vi "Receive and Display using Event Log.vi"() -> ()   [LabVIEW 2023]
uses:
  <instrlib>/BTICardLib/Public/Controls/Event Log Type.ctl
  <instrlib>/BTICardLib/Private/Initialize By Card Number and Core Number.vi
  <instrlib>/BTICardLib/Private/Configure Core From XML.vi
  <instrlib>/BTI429Lib/Private/Rx/Configure/Configure Rx Channel From XML.vi
  <instrlib>/BTI429Lib/Private/Rx/Configure/Get Rx Label Handle Name.vi
  <instrlib>/BTI429Lib/Private/Core/Action-Status/Start Channel.vi
  <instrlib>/BTI429Lib/Private/Core/Action-Status/Stop Channel.vi
  <instrlib>/BTICardLib/BTICardLV.lvlib
  <instrlib>/BTI429Lib/BTI429LV.lvlib
panel:
  out "CoreXml Path":path
  out "Channel Xml Path":path
  in  "Channel number":i32
  in  "core number":i32
  in  "Channel Configuration XML file name":string="Channel Config.xml"
  in  "Core Configuration XML file name":string="Core Config.xml"
  out "error out":errorcluster
  in  "Card Number":i32
  out "Data 2":u32 format="%x"
  out "Data 1":u32 format="%x"
  out "Default":u32 format="%x"
  in  "stop":bool
  # "ARINC 429: Receive Labels"
  # "©2016 Astronics Ballard Technology"
  # "The  message labels are read from the Channel Configuration XML file.\n\nThe label definitions enable Event Log Recording of Message actitivty. The \nEvent Log is polled for 429 Messages and when a specific label has been \nreceived, its data is updated on the front panel."
  # "Always Stop the card\nand Close the card when\ndone. Otherwise, the hardware\ncontinues to operate."
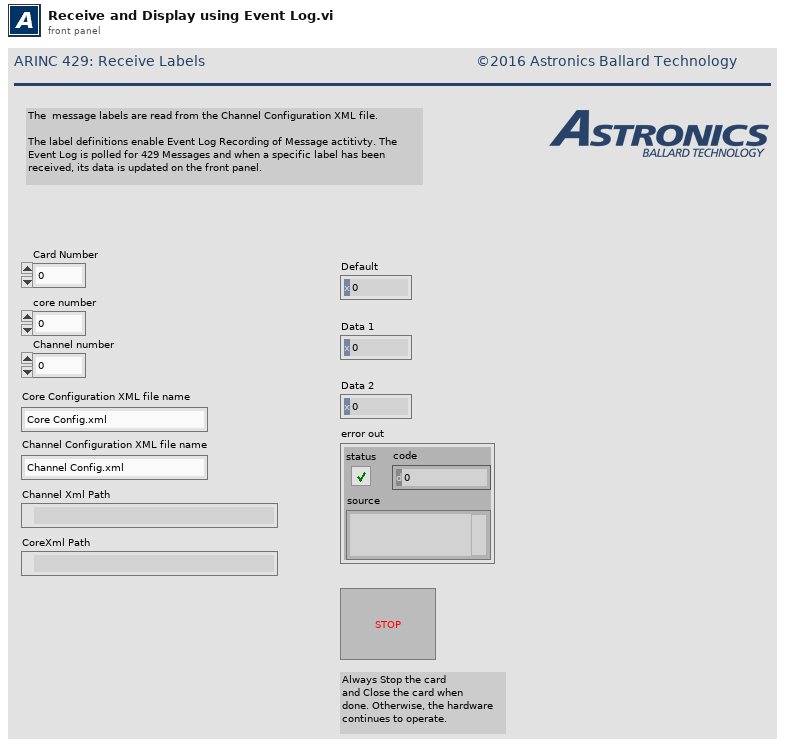
[diagram p1: front panel]
types:
  T1 = typedef "BTICardLV.lvlib/Event Log Type.ctl" = u32
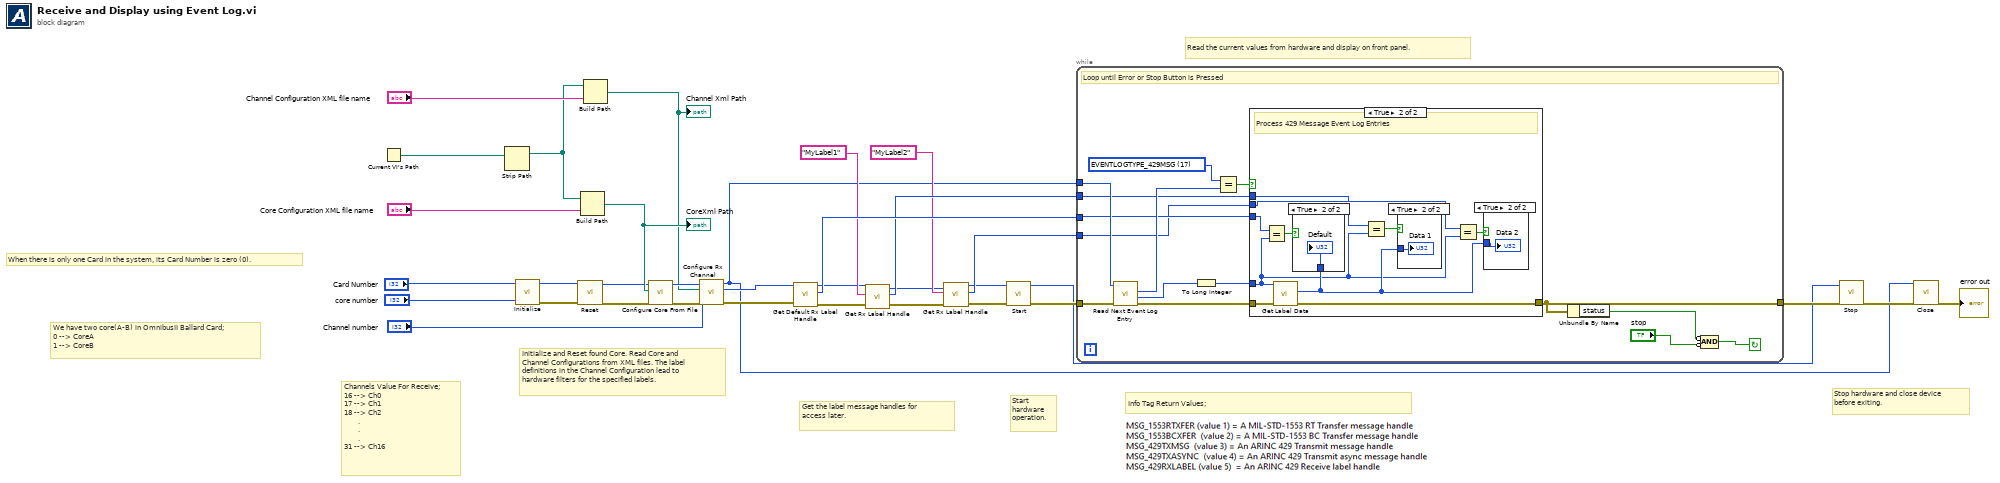
[diagram p0: block diagram]
diagram:
  # "We have two core(A-B) in OmnibusII Ballard Card;\n0 --> CoreA\n1 --> CoreB"
  # "When there is only one Card in the system, its Card Number is zero (0)."
  # "Channels Value For Receive;\n16 --> Ch0\n17 --> Ch1\n18 --> Ch2\n       .\n       .\n       .\n31 --> Ch16"
  # "Info Tag Return Values;"
  # "Stop hardware and close device\nbefore exiting."
  # "Read the current values from hardware and display on front panel."
  # "Start\nhardware\noperation."
  # "Get the label message handles for\naccess later."
  # "Initialize and Reset found Core. Read Core and\nChannel Configurations from XML files. The label\ndefinitions in the Channel Configuration lead to\nhardware filters for the specified labels."
  n1 = Current VI's Path() -> (path=w13:path)
  n2 = Strip Path(path=w13) -> (stripped path=w11:path)  [unwired: 1 out]
  n3 = call-poly <instrlib>:"Initialize.vi"("core number"="core number", "card number"="Card Number") -> ("error out"=w6:errorcluster, "core handle out"=w4:u64)  [unwired: 8 in]
  n4 = call <instrlib>:"Reset.vi"("error in (no error)"=w6, "core handle in"=w4) -> ("error out"=w5:errorcluster, "core handle out"=w3:u64)  [unwired: 8 in]
  n5 = Build Path(base path=w11, name or relative path="Core Configuration XML file name") -> (appended path=w9:path)
  "CoreXml Path" <- w9
  n6 = Build Path(base path=w11, name or relative path="Channel Configuration XML file name") -> (appended path=w8:path)
  "Channel Xml Path" <- w8
  n7 = call-poly <instrlib>:"Configure Core From File.vi"("error in (no error)"=w5, "configuration file path"=w9, "core handle in"=w3) -> ("error out"=w25:errorcluster, "core handle out"=w20:u64)  [unwired: 7 in]
  n8 = call-poly <instrlib>:"Configure Rx Channel.vi"("error in (no error)"=w25, "channel number in"="Channel number", "configuration file path"=w8, "core handle in"=w20) -> ("error out"=w34:errorcluster, "channel handle out"=w19:u64, "core handle out"=w18:u64)  [unwired: 5 in]
  n9 = call <instrlib>:"Get Default Rx Label Handle.vi"("error in (no error)"=w34, "channel handle in"=w19) -> ("error out"=w33:errorcluster, "default label handle out"=w29:u64, "channel handle out"=w17:u64)  [unwired: 7 in]
  n10 = call-poly <instrlib>:"Get Rx Label Handle.vi"("error in (no error)"=w33, "label name"="MyLabel1", "channel handle in"=w17) -> ("error out"=w32:errorcluster, "label handle out"=w28:u64, "channel handle out"=w16:u64)  [unwired: 6 in]
  n11 = call-poly <instrlib>:"Get Rx Label Handle.vi"("error in (no error)"=w32, "label name"="MyLabel2", "channel handle in"=w16) -> ("error out"=w31:errorcluster, "label handle out"=w27:u64, "channel handle out"=w15:u64)  [unwired: 6 in]
  n12 = call-poly <instrlib>:"Start.vi"("error in (no error)"=w31, "channel handle in"=w15) -> ("error out"=w30:errorcluster, "channel handle out"=w14:u64)  [unwired: 8 in]
  n13 = while {
    tunnel: w30 -> [w46]
    tunnel: w29 -> [w40]
    tunnel: w28 -> [w37]
    tunnel: w27 -> [w38]
    tunnel: [w39] -> w21
    tunnel: w18 -> [w44]
    stop <- w49 continue-if-true
    w42 = T1 17 items=["EVENTLOGTYPE_NONE"=0, "EVENTLOGTYPE_1553MSG"=1, "EVENTLOGTYPE_1553OPCODE"=2, "EVENTLOGTYPE_1553HALT"=3, "EVENTLOGTYPE_1553PAUSE"=4, "EVENTLOGTYPE_1553LIST"=5, "EVENTLOGTYPE_1553SERIAL"=6, "EVENTLOGTYPE_429MSG"=17, "EVENTLOGTYPE_429OPCODE"=18, "EVENTLOGTYPE_429HALT"=19, "EVENTLOGTYPE_429PAUSE"=20, "EVENTLOGTYPE_429LIST"=21, "EVENTLOGTYPE_429ERR"=22, "EVENTLOGTYPE_DIOEDGE"=96, "EVENTLOGTYPE_DIOFAULT"=97, "EVENTLOGTYPE_BITERROR"=113] ("x")
    # "Loop until Error or Stop Button is Pressed"
    n14 = call <instrlib>:"Read Next Event Log Entry.vi"("error in (no error)"=w46, "core handle in"=w44) -> ("error out"=w45:errorcluster, "info tag"=w35:u64, "event log entry type"=w43:T1)  [unwired: 4 in, 3 out]
    n15 = To Long Integer(number=w35) -> (32bit integer=w36:i32)
    n16 = Equal?(x=w42, y=w43) -> (x = y?=w41:bool)
    n17 = case shown="True" w41 {
      tunnel: w45 -> [w50 w60]
      tunnel: w36 -> [_ w52]
      tunnel: w40 -> [_ w57]
      tunnel: [w50 w56] -> w39
      tunnel: w38 -> [_ w54]
      tunnel: w37 -> [_ w51]
      frame False {
        # "No 429 Messages to Process"
      }
      frame True {
        # "Process 429 Message Event Log Entries"
        n18 = Equal?(x=w57, y=w52) -> (x = y?=w58:bool)
        n19 = call <instrlib>:"Get Label Data.vi"("error in (no error)"=w60, "label handle in"=w52) -> ("error out"=w56:errorcluster, "value"=w59:u32)  [unwired: 7 in, 1 out]
        n20 = case shown="True" w58 {
          tunnel: w59 -> [_ w61]
          frame False {
          }
          frame True {
            "Default" <- w61
          }
        }
        n21 = Equal?(x=w51, y=w52) -> (x = y?=w53:bool)
        n22 = case shown="True" w53 {
          tunnel: w59 -> [_ w62]
          frame False {
          }
          frame True {
            "Data 1" <- w62
          }
        }
        n23 = Equal?(x=w54, y=w52) -> (x = y?=w55:bool)
        n24 = case shown="True" w55 {
          tunnel: w59 -> [_ w63]
          frame False {
          }
          frame True {
            "Data 2" <- w63
          }
        }
      }
    }
    n25 = Unbundle By Name(w39) -> ("status"=w47:bool)
    n26 = Compound Arithmetic op=AND(invert w47, invert "stop") -> (w49:bool)
  }
  n27 = call-poly <instrlib>:"Stop.vi"("error in (no error)"=w21, "channel handle in"=w14) -> ("error out"=w26:errorcluster)  [unwired: 8 in, 1 out]
  n28 = call <instrlib>:"Close.vi"("error in (no error)"=w26, "core handle in"=w18) -> ("error out"=→"error out":errorcluster)  [unwired: 8 in, 1 out]
